vi "Single Launcher.vi"(8 "error in (no errors)":errorcluster) -> (0 "error out":errorcluster, 3 "Documentation Tool Model":refnum<class "Message Enqueuer.lvclass">)   [LabVIEW 2015]
uses:
  <vilib>/ActorFramework/Actor/Actor.lvclass
  Model/Model.lvclass
  Model Messages/Test Actor Message Msg/Test Actor Message Msg.lvclass
  <vilib>/ActorFramework/Message Enqueuer/Message Enqueuer.lvclass
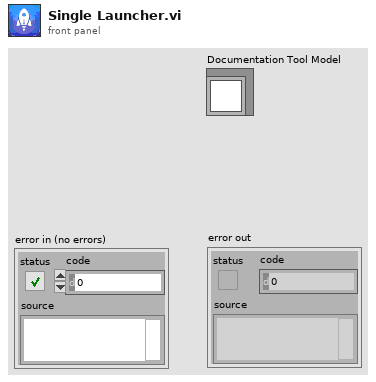
[diagram p1: front panel]
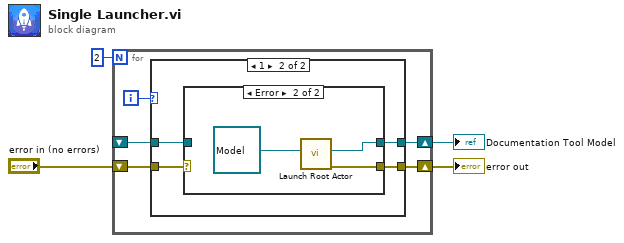
[diagram p0: block diagram]
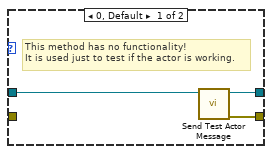
[diagram p2: hidden frame]
diagram:
  n1 = for {
    N: 2 -> [_]
    shift-right: [w8] -> w2
    shift-left: _ -> [w7]
    shift-right: [w6] -> w3
    shift-left: "error in (no errors)" -> [w5]
    i -> [w9]
    n2 = case shown="1" w9 {
      tunnel: [w12 w14] -> w8
      tunnel: w7 -> [w10 w13]
      tunnel: [w11 w15] -> w6
      tunnel: w5 -> [_ w16]
      frame 0, Default {
        # "This method has no functionality!\nIt is used just to test if the actor is working."
        n3 = call "Send Test Actor Message.vi"("Message Enqueuer"=w10) -> ("error out"=w11:errorcluster, "Message Enqueuer out"=w12:refnum<class "Message Enqueuer.lvclass">)  [unwired: 9 in]
      }
      frame 1 {
        n4 = case shown="Error" w16 {
          selector: w16 -> [w17 _]
          tunnel: [w17 w21] -> w15
          tunnel: [w18 w20] -> w14
          tunnel: w13 -> [w18 _]
          frame No Error {
          }
          frame Error {
            n5 = call <vilib>:"Launch Root Actor.vi"("Actor"=refnum<class "Model.lvclass"> refnum ("Model.lvlib:Model.lvclass")) -> ("error out"=w21:errorcluster, "Actor's Enqueuer"=w20:refnum<class "Message Enqueuer.lvclass">)  [unwired: 9 in]
          }
        }
      }
    }
  }
  "Documentation Tool Model" <- w2
  "error out" <- w3
